vi "RS_gen_mod.vi"(8 "Internal Frequency":dbl=1000.0 min=1.0) -> ()   [LabVIEW 2013]
panel:
  in  "Generator":bool
  in  "Refference frequency (MHz)":u16(ring) items=["External", "Internal"]
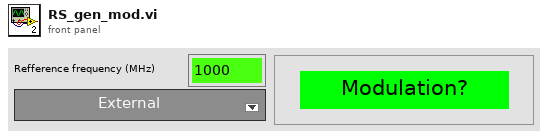
[diagram p1: front panel]
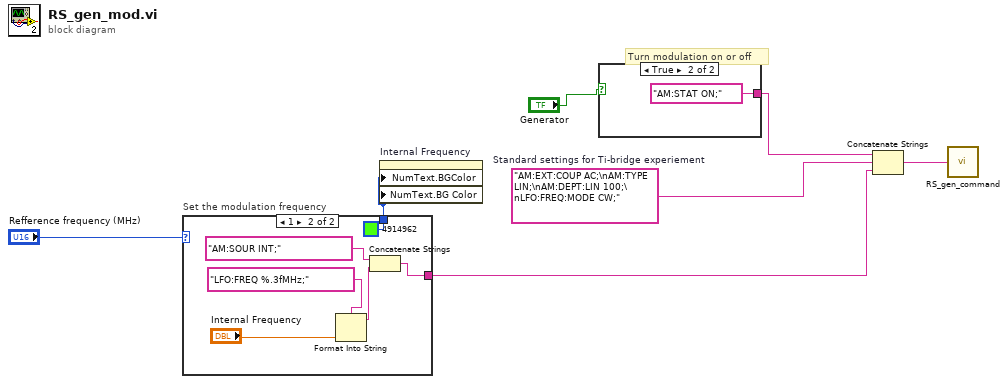
[diagram p0: block diagram]
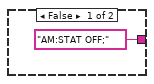
[diagram p2: hidden frame]
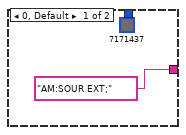
[diagram p3: hidden frame]
diagram:
  w4 = "AM:EXT:COUP AC;\nAM:TYPE LIN;\nAM:DEPT:LIN 100;\nLFO:FREQ:MODE CW;"  # Standard settings for Ti-bridge experiement
  # "Turn modulation on or off"
  n1 = case "Set the modulation frequency" shown="1" "Refference frequency (MHz)" {
    tunnel: [u32 7171437 u32 4914962] -> w6
    tunnel: ["AM:SOUR EXT;" ("Comand") w10] -> w2
    frame 0, Default {
    }
    frame 1 {
      n2 = Format Into String(format string="LFO:FREQ %.3fMHz;" ("Comand"), "Internal Frequency") -> (resulting string=w11:string)  [unwired: 2 in, 1 out]
      n3 = Concatenate Strings("AM:SOUR INT;" ("Comand"), w11) -> (w10:string)
    }
  }
  n4 = property on="Internal Frequency" class="DigNum (strict)"("NumText.BGColor"=w6, "NumText.BG Color"=w6) -> ()  [unwired: 2 in, 2 out]
  n5 = case shown="True" "Generator" {
    tunnel: ["AM:STAT OFF;" ("Comand") "AM:STAT ON;" ("Comand")] -> w5
    frame False {
    }
    frame True {
    }
  }
  n6 = Concatenate Strings(w5, w4, w2) -> (w3:string)
  n7 = call "RS_gen_command.vi"("Comand"=w3) -> ()  [unwired: 4 in, 1 out]
